vi "Items In Range.vi"(10 "Location Translation":cluster{"dst":i64, "src":i64, "rng":i64}, 11 "Initial Items":cluster{"strt":i64, "rng":i64}) -> (2 "Keep?":bool, 3 "Items In Range":cluster{i64, "upper limit":i64})   [LabVIEW 2023, in "d5.lvlib"]
uses:
  d5.lvlib
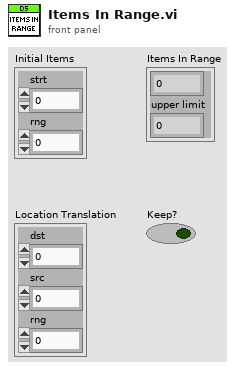
[diagram p1: front panel]
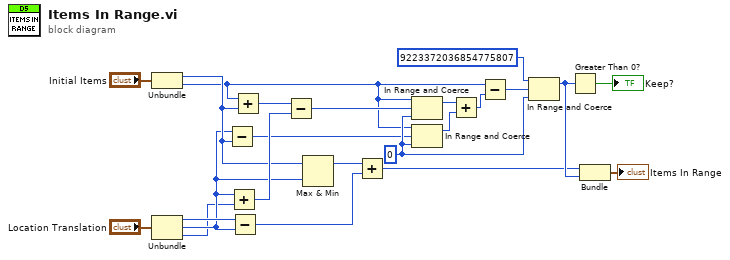
[diagram p0: block diagram]
diagram:
  w10 = i64 0 ("x")
  n1 = Unbundle("Initial Items") -> ("strt"=w6:i64, "rng"=w5:i64)
  n2 = Unbundle("Location Translation") -> ("dst"=w4:i64, "src"=w3:i64, "rng"=w2:i64)
  n3 = Subtract(x=w3, y=w6) -> (x-y=w9:i64)
  n4 = Add(x=w3, y=w2) -> (x+y=w20:i64)
  n5 = Subtract(x=w4, y=w3) -> (x-y=w18:i64)
  n6 = Add(x=w5, y=w6) -> (x+y=w8:i64)
  n7 = Subtract(x=w8, y=w20) -> (x-y=w7:i64)
  n8 = Max & Min(x=w6, y=w3) -> (max(x,y)=w17:i64)  [unwired: 1 out]
  n9 = Add(x=w17, y=w18) -> (x+y=w1:i64)
  n10 = In Range and Coerce(upper limit=w5, x=w7, lower limit=w10) -> (coerced(x)=w16:i64)  [unwired: 1 out]
  n11 = In Range and Coerce(upper limit=w5, x=w9, lower limit=w10) -> (coerced(x)=w21:i64)  [unwired: 1 out]
  n12 = Add(x=w16, y=w21) -> (x+y=w11:i64)
  n13 = Subtract(x=w5, y=w11) -> (x-y=w12:i64)
  n14 = In Range and Coerce(upper limit=i64 9223372036854775807, x=w12, lower limit=w10) -> (coerced(x)=w14:i64)  [unwired: 1 out]
  n15 = Greater Than 0?(x=w14) -> (x > 0?=→"Keep?":bool)
  n16 = Bundle(w1, "upper limit"=w14) -> (→"Items In Range":cluster{i64, "upper limit":i64})  [unwired: 1 in]
